vi "get_spectrum-v2.vi"(8 "error in":errorcluster, 10 "Average":i32, 11 "Integration Time (us)":i32) -> (0 "error out":errorcluster, 2 "Spectrum":dbl[](array[numeric]), 3 "Wavelength (nm)":dbl[](array[numeric]))   [LabVIEW 2021]
doc: "André Romero - 2024\nandretec@ifsc.usp.br"
uses:
  <vilib>/Analysis/baseanly.llb/Mean (DBL).vi
  Global_v20.vi
  <instrlib>/Ocean Optics 2000 4000/Ocean Optics 2000 4000.lvlib
  <vilib>/Analysis/NI_AALBase.lvlib
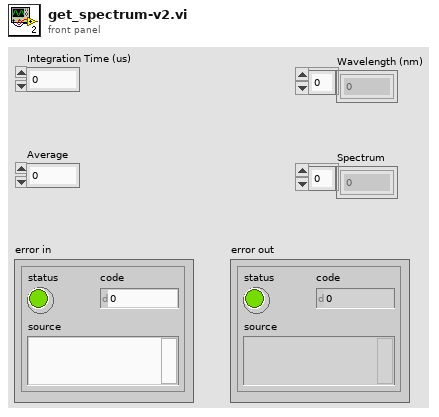
[diagram p1: front panel]
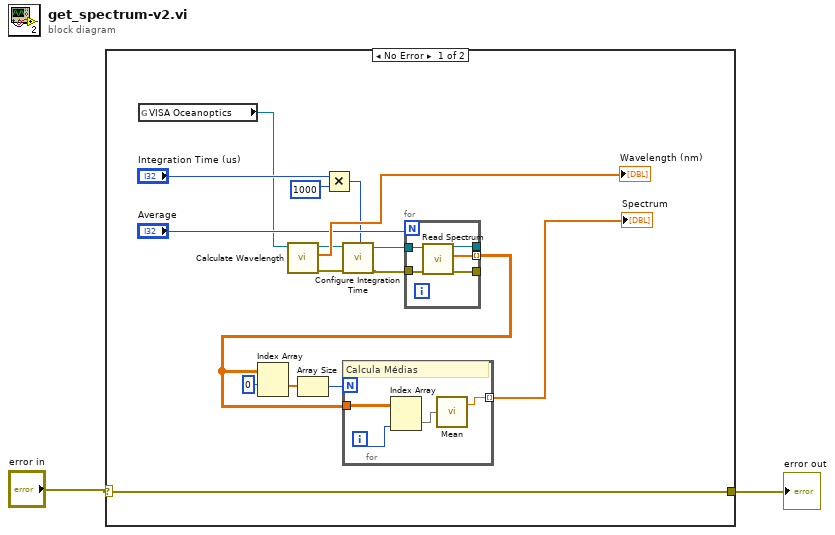
[diagram p0: block diagram]
diagram:
  n1 = case shown="No Error" "error in" {
    selector: "error in" -> [w3 w28]
    tunnel: [w3 w28] -> w1
    frame No Error {
      n2 = global read "Global_v20.vi" "VISA Oceanoptics"() -> (w4:refnum<visa-resource-name>)
      n3 = call <instrlib>:"Calculate Wavelength.vi"("VISA resource name"=w4) -> ("error out"=w6:errorcluster, "Wavelength (nm)"=→"Wavelength (nm)":dbl[], "VISA resource name out"=w7:refnum<visa-resource-name>)  [unwired: 2 in, 6 out]
      n4 = Multiply(x="Integration Time (us)", y=1000) -> (x*y=w8:i32)
      n5 = call <instrlib>:"Configure Integration Time.vi"("error in (no error)"=w6, "Integration Time (6000)"=w8, "VISA resource name"=w7) -> ("error out"=w13:errorcluster, "VISA resource name out"=w14:refnum<visa-resource-name>)  [unwired: 7 in]
      n6 = for {
        N: "Average" -> [_]
        tunnel: w14 -> [w23]
        tunnel: w13 -> [w22]
        tunnel: [w21] -> w16 mode=indexing
        tunnel: [w20] -> _
        tunnel: [w19] -> _
        n7 = call <instrlib>:"Read Spectrum.vi"("error in (no error)"=w22, "VISA resource name"=w23) -> ("error out"=w19:errorcluster, "Spectrum by Pixel Number"=w21:dbl[], "VISA resource name out"=w20:refnum<visa-resource-name>)  [unwired: 6 in, 1 out]
      }
      n8 = Index Array(array=w16, index (row)=0) -> (element=w11:dbl[])  [unwired: 1 in]
      n9 = Array Size(array=w11) -> (size(s)=w12:i32)
      n10 = for {
        N: w12 -> [_]
        tunnel: w16 -> [w27]
        tunnel: [w24] -> w18 mode=indexing
        i -> [w26]
        # "Calcula Médias"
        n11 = Index Array(array=w27, index (col)=w26) -> (element=w25:dbl[])  [unwired: 1 in]
        n12 = call-poly <vilib>:"Mean.vi"("X"=w25) -> ("mean"=w24:dbl)  [unwired: 1 out]
      }
      "Spectrum" <- w18
    }
    frame Error {
    }
  }
  "error out" <- w1
